vi "test - Is Deployed File Newer - 1.vi"(8 "error in (no error)":errorcluster, 11 "TestCase in":refnum<class "Post Build Action Tester.lvclass">) -> (0 "error out":errorcluster, 3 "TestCase out":refnum<class "Post Build Action Tester.lvclass">)   [LabVIEW 2016, in "Post Build Action Tester.lvclass"]
uses:
  Post Build Action Tester.lvclass
  <vilib>/addons/_JKI Toolkits/VI Tester/TestCase.llb/TestCase.lvclass
  C:/Program Files (x86)/National Instruments/LabVIEW 2016/vi.lib/addons/_JKI Toolkits/VI Tester/TestCase.llb/TestCase.lvclass
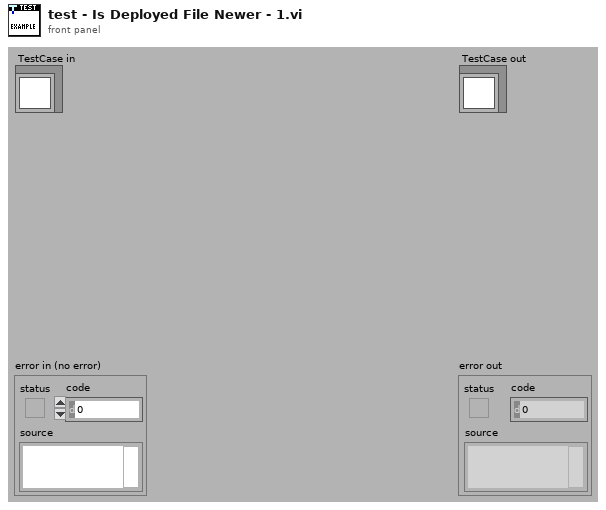
[diagram p1: front panel]
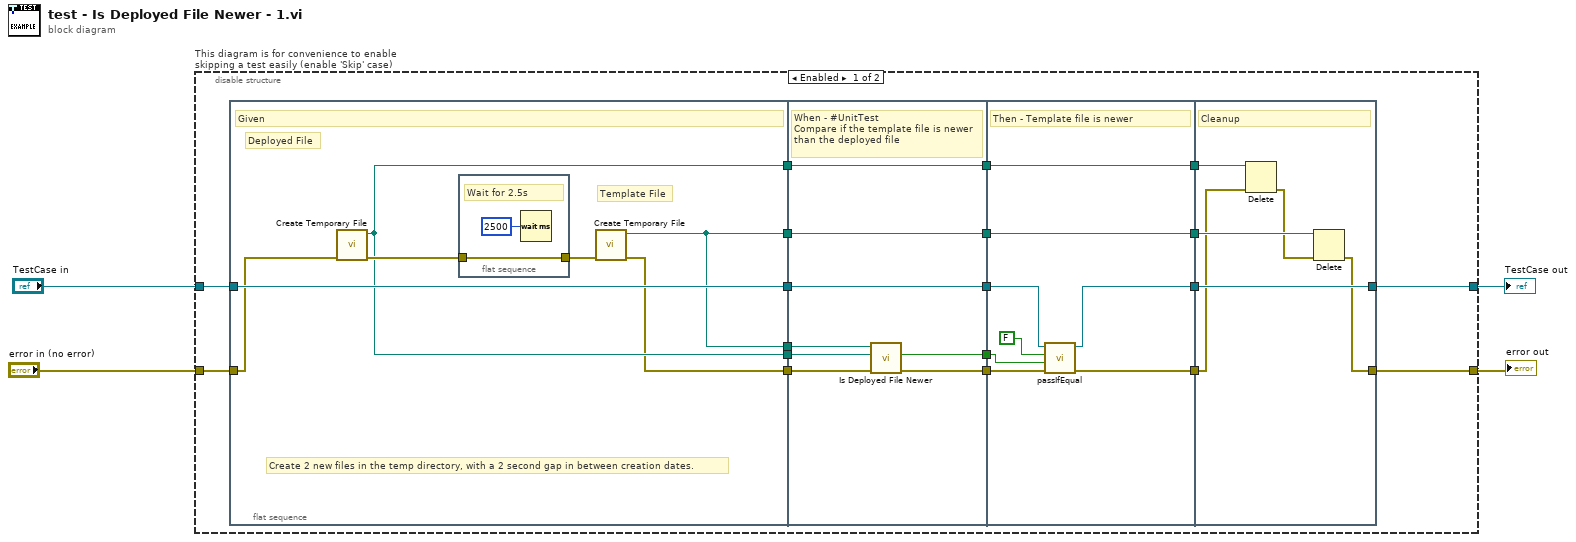
[diagram p0: block diagram]
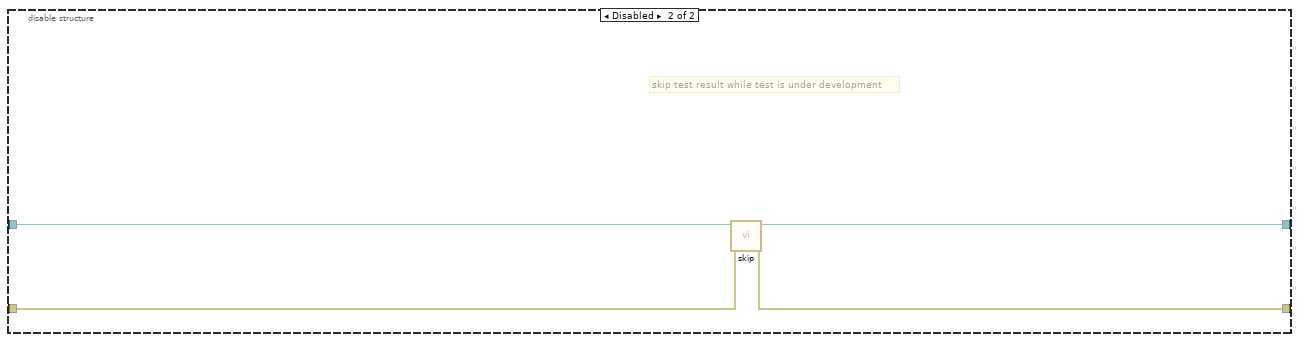
[diagram p2: hidden frame]
diagram:
  n1 = disable-structure "This diagram is for convenience to enable skipping a test easily (enable 'Skip' case)" shown="Enabled" {
    disable-tunnel: "TestCase in" -> [w16 w58]
    disable-tunnel: [w15 w56] -> w1
    disable-tunnel: [w14 w57] -> w3
    disable-tunnel: "error in (no error)" -> [w17 w55]
    frame Enabled {
      n2 = flat-sequence {
        tunnel: w17 -> [w29]
        tunnel: w16 -> [w30]
        tunnel: [w30] -> w23
        tunnel: [w25] -> w22
        tunnel: [w27] -> w11
        tunnel: [w24] -> w8
        tunnel: [w24] -> w7
        tunnel: [w27] -> w5
        tunnel: [w40] -> w21
        tunnel: [w36] -> w20
        tunnel: w23 -> [w40]
        tunnel: w22 -> [w39]
        tunnel: [w38] -> w12
        tunnel: w11 -> [w38]
        tunnel: [w37] -> w9
        tunnel: w8 -> [w37]
        tunnel: w7 -> [w35]
        tunnel: [w33] -> w6
        tunnel: w5 -> [w34]
        tunnel: [w47] -> w19
        tunnel: [w45] -> w18
        tunnel: w21 -> [w48]
        tunnel: w20 -> [w46]
        tunnel: [w44] -> w13
        tunnel: w12 -> [w44]
        tunnel: [w43] -> w10
        tunnel: w9 -> [w43]
        tunnel: w6 -> [w42]
        tunnel: [w49] -> w14
        tunnel: [w54] -> w15
        tunnel: w19 -> [w54]
        tunnel: w18 -> [w51]
        tunnel: w13 -> [w53]
        tunnel: w10 -> [w52]
        frame #0 {
          # "Template File"
          # "Deployed File"
          # "Create 2 new files in the temp directory, with a 2 second gap in between creation dates."
          # "Given"
          n3 = call "Create Temporary File.vi"("error in (no error)"=w29) -> ("error out"=w28:errorcluster, "Temp file path"=w27:path)  [unwired: 9 in]
          n4 = flat-sequence {
            tunnel: w28 -> [w32]
            tunnel: [w32] -> w26
            frame #0 {
              # "Wait for 2.5s"
              n5 = Wait (ms)(milliseconds to wait=u32 2500) -> ()  [unwired: 1 out]
            }
          }
          n6 = call "Create Temporary File.vi"("error in (no error)"=w26) -> ("error out"=w25:errorcluster, "Temp file path"=w24:path)  [unwired: 9 in]
        }
        frame #1 {
          # "When - #UnitTest\nCompare if the template file is newer than the deployed file"
          n7 = call "Is Deployed File Newer.vi"("error in (no error)"=w39, "Deployed Path"=w34, "Template Path"=w35) -> ("error out"=w36:errorcluster, "Deployed Newer?"=w33:bool)  [unwired: 7 in]
        }
        frame #2 {
          # "Then - Template file is newer"
          n8 = call-dynamic "passIfEqual.vi"("error in (no error)"=w46, "y"=w42, "x"=FALSE, "TestCase in"=w48) -> ("error out"=w45:errorcluster, "TestCase out"=w47:refnum<class "Post Build Action Tester.lvclass">)  [unwired: 6 in]
        }
        frame #3 {
          # "Cleanup"
          n9 = Delete(path (use dialog)=w53, error in=w51) -> (error out=w50:errorcluster)  [unwired: 3 in, 2 out]
          n10 = Delete(path (use dialog)=w52, error in=w50) -> (error out=w49:errorcluster)  [unwired: 3 in, 2 out]
        }
      }
    }
    frame Disabled {
      # "skip test result while test is under development"
      n11 = call <vilib>:"skip.vi"("error in (no error)"=w55, "TestCase in"=w58) -> ("error out"=w57:errorcluster, "TestCase out"=w56:refnum<class "Post Build Action Tester.lvclass">)  [unwired: 8 in]
    }
  }
  "error out" <- w3
  "TestCase out" <- w1
